vi "Mac_Get Font Name Array.vi"(8 "error in (no error)":errorcluster) -> (0 "error out":errorcluster, 3 "Array":string[](array[string]))   [LabVIEW 2021]
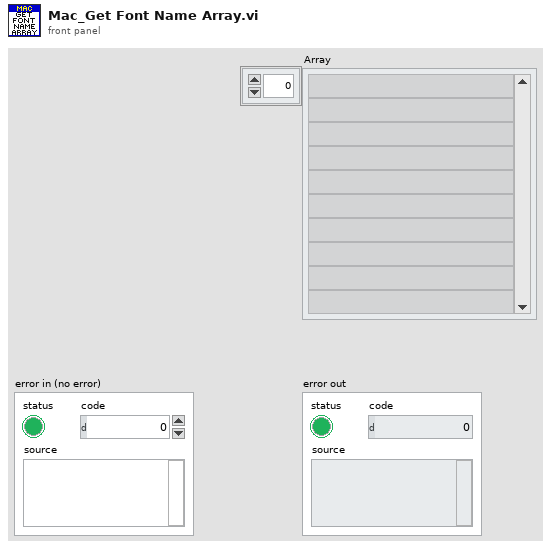
[diagram p1: front panel]
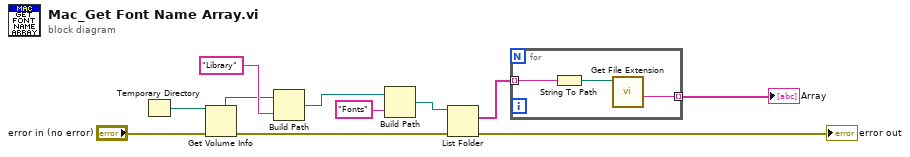
[diagram p0: block diagram]
diagram:
  n1 = Temporary Directory() -> (w2:path)
  n2 = Get Volume Info(8:"error in (no error)", 11:w2) -> (0:w9:errorcluster, 5:w3:path)  [unwired: 4 out]
  n3 = Build Path(base path=w3, name or relative path="Library") -> (appended path=w6:path)
  n4 = Build Path(base path=w6, name or relative path="Fonts") -> (appended path=w8:path)
  n5 = List Folder(path=w8, error in=w9) -> (filenames=w10:string[], error out=→"error out":errorcluster)  [unwired: 4 out]
  n6 = for {
    tunnel: w10 -> [w14] mode=indexing
    tunnel: [w12] -> w1 mode=indexing
    n7 = String To Path(string=w14) -> (path=w13:path)
    n8 = call <vilib>:"Get File Extension.vi"("file"=w13) -> ("filename without extension"=w12:string)  [unwired: 1 in, 9 out]
  }
  "Array" <- w1
